vi "Contraseñas.vi"(11 "String":string) -> (3 "Contraseña Correcta?":bool)   [LabVIEW 2017]
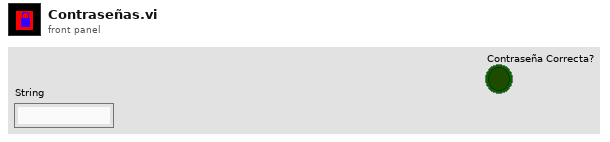
[diagram p1: front panel]
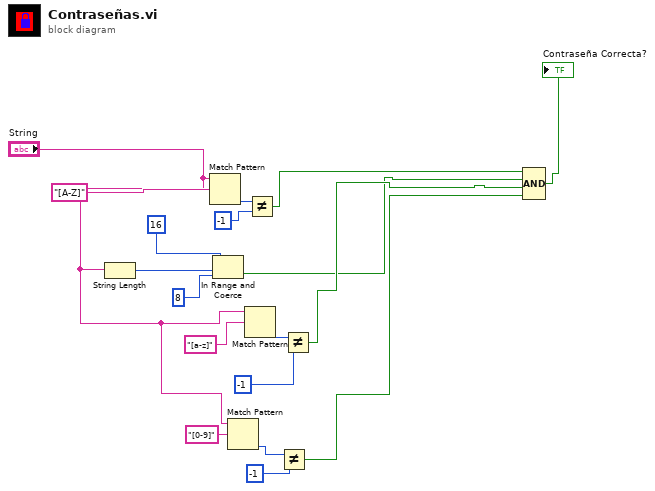
[diagram p0: block diagram]
diagram:
  n1 = String Length(string="String") -> (length=w5:i32)
  n2 = Match Pattern(string="String", regular expression="[A-Z]") -> (offset past match=w17:i32)  [unwired: 1 in, 3 out]
  n3 = In Range and Coerce(upper limit=16, x=w5, lower limit=8) -> (In Range?=w6:bool)  [unwired: 1 out]
  n4 = Match Pattern(string="String", regular expression="[0-9]") -> (offset past match=w11:i32)  [unwired: 1 in, 3 out]
  n5 = Match Pattern(string="String", regular expression="[a-z]") -> (offset past match=w14:i32)  [unwired: 1 in, 3 out]
  n6 = Not Equal?(x=w17, y=-1) -> (x != y?=w7:bool)
  n7 = Not Equal?(x=w11, y=-1) -> (x != y?=w9:bool)
  n8 = Not Equal?(x=w14, y=-1) -> (x != y?=w10:bool)
  n9 = Compound Arithmetic op=AND(w7, w6, w10, w9) -> (→"Contraseña Correcta?":bool)
